vi "DataColumnHead.vi"(8 "error in (no error)":errorcluster caption="错误输入（无错误）", 11 "TPlot 输入":refnum<class "TPlot.lvclass">) -> (0 "error out":errorcluster caption="错误输出", 2 "首行":string[](array[string]), 3 "TPlot 输出":refnum<class "TPlot.lvclass">)   [LabVIEW 2018, in "DataDisplay.lvlib" / "TPlot.lvclass"]
uses:
  TPlot.lvclass
  TPlot.lvclass/TPlot.ctl
  SubVI/DD_Parameter.vi
  DataDisplay.lvlib
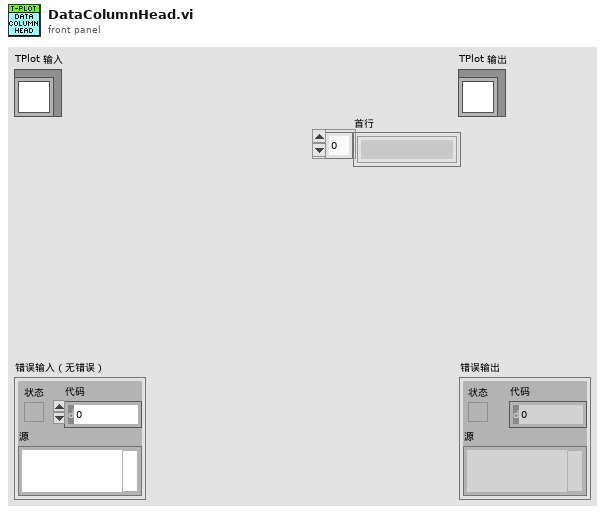
[diagram p1: front panel]
types:
  T1 = typedef "DataDisplay.lvlib/DD_ChannelInfo.ctl" = cluster{"名称":string, "单位":string, "数据类型":enum16{"Real", "Int"}, "趋势线":enum16{"N/A", "X", "Y"}}
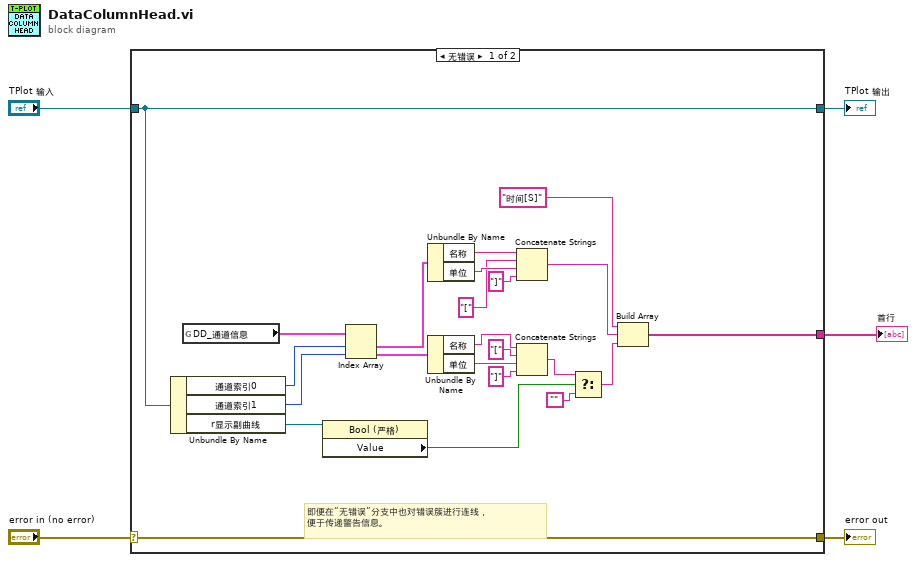
[diagram p0: block diagram]
diagram:
  n1 = case shown="无错误" "error in (no error)" {
    selector: "error in (no error)" -> [w28 w30]
    tunnel: [w28 w30] -> w4
    tunnel: [w27 w29] -> w2
    tunnel: "TPlot 输入" -> [w27 w29]
    tunnel: [w12 _] -> w1
    frame No Error {
      # "即便在“无错误”分支中也对错误簇进行连线，\n便于传递警告信息。"
      n2 = Unbundle By Name(w27) -> ("通道索引0"=w25:i32, "通道索引1"=w24:i32, "r显示副曲线"=w10:refnum<vi>)
      n3 = global read "DD_Parameter.vi" "DD_通道信息"() -> (w26:T1[])
      n4 = property class="Bool (严格)"(reference=w10) -> ("Value"=w8:bool)  [unwired: 1 in, 2 out]
      n5 = Index Array(array=w26, index #1=w25, index #2=w24) -> (element #1=w23:T1, element #2=w18:T1)
      n6 = Unbundle By Name(w23) -> ("名称"=w22:string, "单位"=w21:string)
      n7 = Unbundle By Name(w18) -> ("名称"=w11:string, "单位"=w15:string)
      n8 = Concatenate Strings(w22, "[" ("字符串"), w21, "]" ("字符串")) -> (w13:string)
      n9 = Concatenate Strings(w11, "[" ("字符串"), w15, "]" ("字符串")) -> (w9:string)
      n10 = Select(t=w9, s=w8, f="") -> (s? t:f=w6:string)
      n11 = Build Array("时间[S]", w13, w6) -> (w12:string[])
    }
    frame Error {
    }
  }
  "error out" <- w4
  "TPlot 输出" <- w2
  "首行" <- w1
